vi "Teleop.vi"(10 "Match Info":T1={"Autonomous Elapsed Seconds"=0.0, "TeleOp Elapsed Seconds"=0.0, "Disabled Elapsed Seconds"=0.0, "Visited Autonomous"=FALSE, "Visited TeleOp"=FALSE, "Visited Disabled"=FALSE, "Autonomous Settings"={"Autonomous Style"=enum."Independent", "VI Refnum"=refnum}}, 11 "Call Context":T2) -> ()   [LabVIEW 2011]
doc: "This VI is called for each TeleOp packet received from the DS where the robot is not disabled. It is often used to read from the joysticks and update I/O or to update setpoints for timed control loops. It should complete and return within 20 milliseconds or it may miss DS packets."
uses:
  <vilib>/Rock Robotics/WPI/DriverStation/WPI_DriverStationDerivedRobotMode.ctl
  <vilib>/Rock Robotics/WPI/DriverStation/WPI_DriverStationMatch Info.ctl
  <vilib>/Rock Robotics/WPI/Relay/WPI_RelayValue.ctl
  <vilib>/Rock Robotics/WPI/DriverStation/DriverStationLCD/WPI_DriverStationLCDLCDLine.ctl
  Robot Global Data.vi
panel:
  in  "LDrive0":dbl
  in  "Rdrive0":dbl=0.9
  in  "Rdrive2":dbl=0.6
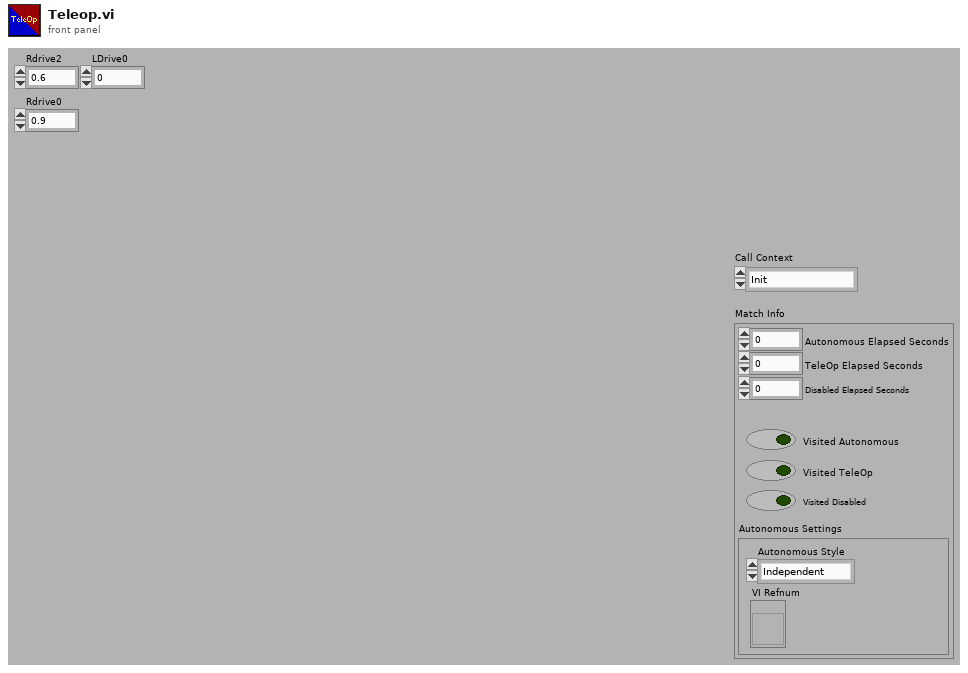
[diagram p1: front panel]
types:
  T1 = typedef "WPI_DriverStationMatch Info.ctl" = cluster{"Autonomous Elapsed Seconds":dbl, "TeleOp Elapsed Seconds":dbl, "Disabled Elapsed Seconds":dbl, "Visited Autonomous":bool, "Visited TeleOp":bool, "Visited Disabled":bool, "Autonomous Settings":cluster{"Autonomous Style":enum16{"Iterative", "Independent"}, "VI Refnum":refnum<vi>}}
  T2 = typedef "WPI_DriverStationDerivedRobotMode.ctl" = enum16{"Init", "Execute", "Stop"}
  T3 = typedef "WPI_RelayValue.ctl" = enum16{"Off", "On", "Forward", "Reverse"}
  T4 = typedef "WPI_JoystickDevRef.ctl" = cluster{"Device":T5}
  T5 = typedef "WPI_JoystickDeviceEnum.ctl" = enum16{"USB 1", "USB 2", "USB 3", "USB 4", "Kinect 1", "Kinect 2"}
  T6 = typedef "WPI_JoystickButtonState.ctl" = cluster{"Button 1":bool, "Button 2":bool, "Button 3":bool, "Button 4":bool, "Button 5":bool, "Button 6":bool, "Button 7":bool, "Button 8":bool, "Button 9":bool, "Button 10":bool, "Button 11":bool, "Button 12":bool}
  T7 = cluster{"axis 1 (x)":dbl, "axis 2 (y)":dbl, "axis 3 (throttle)":dbl, "axis 4":dbl, "axis 5":dbl, "axis 6":dbl}
  T8 = typedef "WPI_MotorControlDeviceRef.ctl" = cluster{"DeviceStatus":errorcluster, "Type":enum16{"PWM", "CAN"}, "PWM":cluster{"Digital Module":T9, "PWM Channel":T10, "DeadBand":T11}, "CAN":cluster{"Device Number":u8, "Control Mode":T12, "Semaphore":T13, "Max Vout":dbl}, "Invert":bool, "TransformRef":T14, "InvTransformRef":T14}
  T9 = typedef "FPGA_TypedefDigitalModule.ctl" = enum16{"Digital Module 1", "Digital Module 2"}
  T10 = typedef "FPGA_DIOPWMChannel.ctl" = enum8{"PWM 1", "PWM 2", "PWM 3", "PWM 4", "PWM 5", "PWM 6", "PWM 7", "PWM 8", "PWM 9", "PWM 10", "Invalid"}
  T11 = typedef "WPI_PWMDeadband.ctl" = cluster{"Name":string, "maxPositivePwm":i32, "minPositivePwm":i32, "centerPwm":i32, "maxNegativePwm":i32, "minNegativePwm":i32, "angularRange":u16}
  T12 = typedef "WPI_CANJaguar_ControlMode.ctl" = enum8{"Percent VBus", "Current", "Speed", "Position", "Voltage"}
  T13 = typedef "Semaphore RefNum" = refnum<k1>
  T14 = typedef "WPI_PWMTransform_ConPane.ctl" = refnum<vi>
  T15 = cluster{"Driver Station Digital Input (1-8)[0]":bool, "Driver Station Digital Input (1-8)[1]":bool, "Driver Station Digital Input (1-8)[2]":bool, "Driver Station Digital Input (1-8)[3]":bool, "Driver Station Digital Input (1-8)[4]":bool, "Driver Station Digital Input (1-8)[5]":bool, "Driver Station Digital Input (1-8)[6]":bool, "Driver Station Digital Input (1-8)[7]":bool, "Driver Station Digital Input (1-8)[8]":bool}
  T16 = typedef "WPI_RelayDevRef.ctl" = cluster{"DevStatus":errorcluster, "Relay Channel":T17, "Digital Module":T9, "Relay Direction":T18}
  T17 = typedef "FPGA_DIORelayChannel.ctl" = enum8{"Relay 1", "Relay 2", "Relay 3", "Relay 4", "Relay 5", "Relay 6", "Relay 7", "Relay 8", "Invalid"}
  T18 = typedef "WPI_RelayDirection.ctl" = enum16{"Both directions", "Forward only", "Reverse only"}
  T19 = typedef "WPI_DigitalInputDevRef.ctl" = cluster{"DevStatus":errorcluster, "DIO Channel":T20, "Digital Module":T9}
  T20 = typedef "FPGA_DIOChannel.ctl" = enum8{"DIO 1", "DIO 2", "DIO 3", "DIO 4", "DIO 5", "DIO 6", "DIO 7", "DIO 8", "DIO 9", "DIO 10", "DIO 11", "DIO 12", "DIO 13", "DIO 14", "Invalid"}
  T21 = typedef "WPI_EncoderDevRef.ctl" = cluster{"DevStatus":errorcluster, "EncoderIndex":T22, "CounterIndex":T23, "DistancePerCount":dbl, "Decoding Type":T24}
  T22 = typedef "FPGA_EncoderIdx.ctl" = enum8{"Enc 0", "Enc 1", "Enc 2", "Enc 3", "Invalid"}
  T23 = typedef "FPGA_CounterCtrSystemIndex.ctl" = enum8{"Ctr 0", "Ctr 1", "Ctr 2", "Ctr 3", "Ctr 4", "Ctr 5", "Ctr 6", "Ctr 7", "Invalid"}
  T24 = typedef "WPI_EncoderType.ctl" = enum16{"1x", "2x", "4x"}
  T25 = typedef "WPI_DriverStationLCDLCDLine.ctl" = enum16{"Main - Line 1", "User - Line 2", "User - Line 3", "User - Line 4", "User - Line 5", "User - Line 6"}
  T26 = typedef "WPI_ServoDeviceRef.ctl" = cluster{"DeviceStatus":errorcluster, "Digital Module":T9, "PWM Channel":T10, "DeadBand":T11}
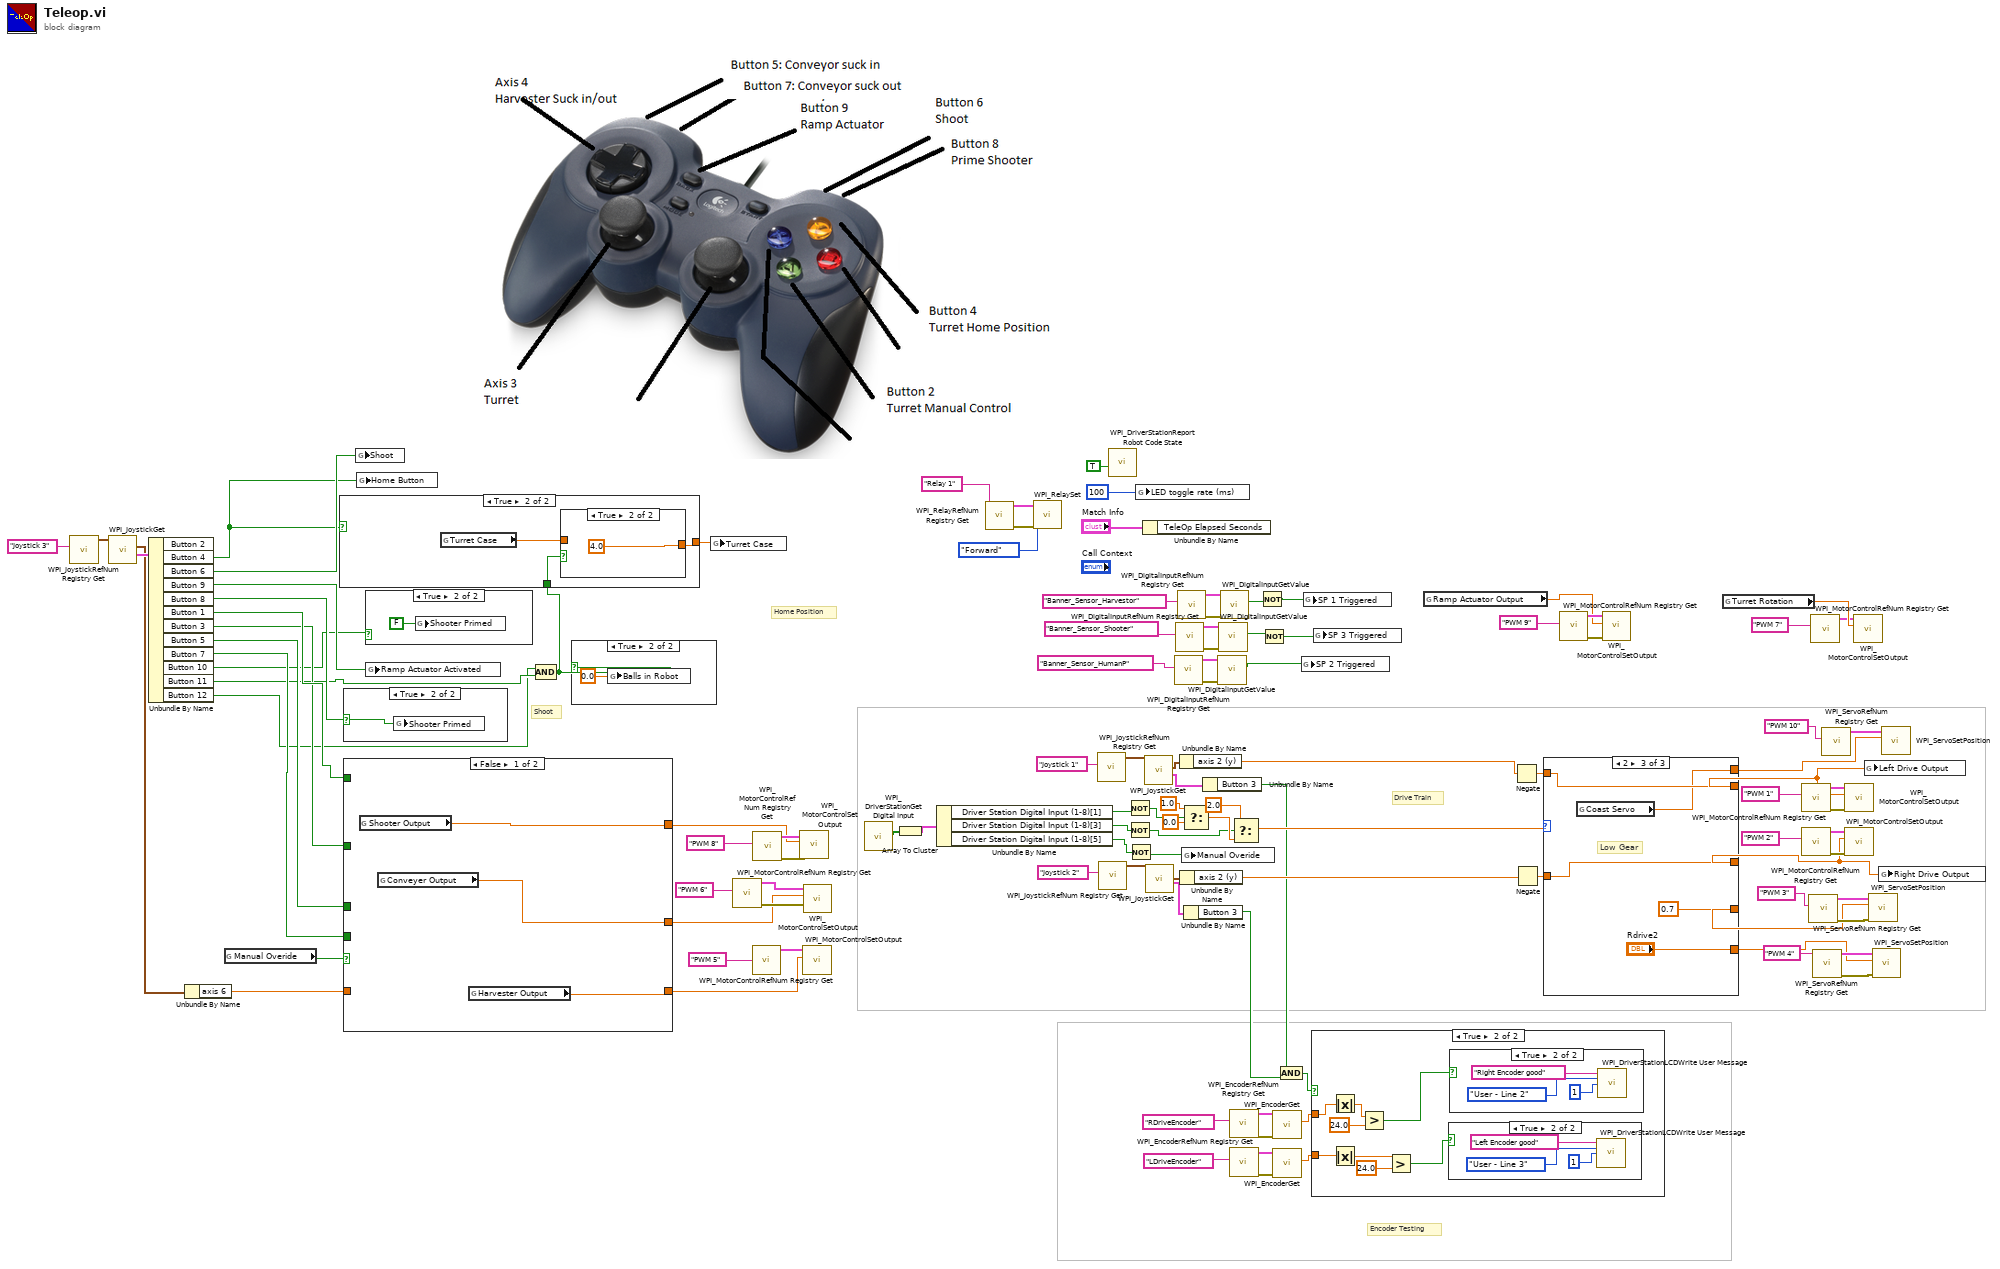
[diagram p0: block diagram]
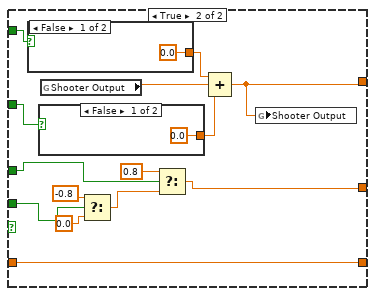
[diagram p7: hidden frame]
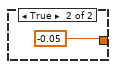
[diagram p8: hidden frame]
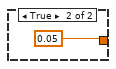
[diagram p9: hidden frame]
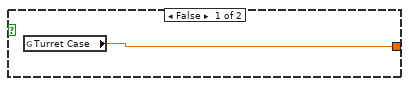
[diagram p11: hidden frame]
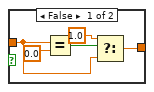
[diagram p12: hidden frame]
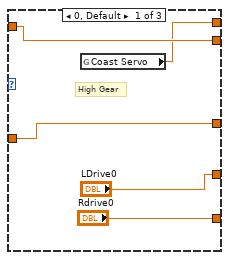
[diagram p13: hidden frame]
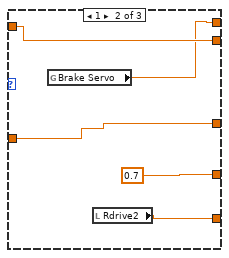
[diagram p14: hidden frame]
diagram:
  # "Encoder Testing"
  # "Shoot"
  # "Home Position"
  # "Drive Train"
  n1 = call <vilib>:"WPI_JoystickRefNum Registry Get.vi"("refnum name"="Joystick 3") -> ("JoystickDevRef"=w66:T4)  [unwired: 9 in, 1 out]
  n2 = call <vilib>:"WPI_JoystickGet.vi"("JoystickDevRef"=w66) -> ("Buttons"=w67:T6, "Axes"=w40:T7)  [unwired: 4 in, 1 out]
  n3 = Unbundle By Name(w67) -> ("Button 4"=w25:bool, "Button 6"=w65:bool, "Button 9"=w69:bool, "Button 8"=w41:bool, "Button 1"=w27:bool, "Button 3"=w26:bool, "Button 5"=w35:bool, "Button 7"=w34:bool, "Button 10"=w24:bool, "Button 11"=w23:bool, "Button 12"=w22:bool)  [unwired: 1 out]
  n4 = Unbundle By Name(w40) -> ("axis 6"=w20:dbl)
  n5 = global read "Robot Global Data.vi" "Manual Overide"() -> (w29:bool)
  n6 = case shown="True" w41 {
    selector: w41 -> [_ w114]
    frame False {
    }
    frame True {
      n7 = global write "Robot Global Data.vi" "Shooter Primed"(w114) -> ()
    }
  }
  n8 = case shown="False" w29 {
    tunnel: [w117 w119] -> w36
    tunnel: w27 -> [_ w124]
    tunnel: w26 -> [_ w123]
    tunnel: w35 -> [_ w126]
    tunnel: w34 -> [_ w127]
    tunnel: [w116 w125] -> w30
    tunnel: [w115 w118] -> w21
    tunnel: w20 -> [_ w118]
    frame False {
      n9 = global read "Robot Global Data.vi" "Shooter Output"() -> (w117:dbl)
      n10 = global read "Robot Global Data.vi" "Conveyer Output"() -> (w116:dbl)
      n11 = global read "Robot Global Data.vi" "Harvester Output"() -> (w115:dbl)
    }
    frame True {
      n12 = case shown="False" w124 {
        tunnel: [0.0 0.05] -> w122
        frame False {
        }
        frame True {
        }
      }
      n13 = case shown="False" w123 {
        tunnel: [0.0 -0.05] -> w121
        frame False {
        }
        frame True {
        }
      }
      n14 = global read "Robot Global Data.vi" "Shooter Output"() -> (w120:dbl)
      n15 = Select(t=-0.8, s=w127, f=0.0) -> (s? t:f=w131:dbl)
      n16 = Select(t=0.8, s=w126, f=w131) -> (s? t:f=w125:dbl)
      n17 = Compound Arithmetic op=ADD(w122, w120, w121) -> (w119:dbl)
      n18 = global write "Robot Global Data.vi" "Shooter Output"(w119) -> ()
    }
  }
  n19 = global write "Robot Global Data.vi" "Shoot"(w65) -> ()
  n20 = global write "Robot Global Data.vi" "Home Button"(w25) -> ()
  n21 = case shown="True" w24 {
    frame False {
    }
    frame True {
      n22 = global write "Robot Global Data.vi" "Shooter Primed"(FALSE ("Shooter Primed")) -> ()
    }
  }
  n23 = global write "Robot Global Data.vi" "Ramp Actuator Activated"(w69) -> ()
  n24 = Compound Arithmetic op=AND(w22, w23) -> (w19:bool)
  n25 = case shown="True" w25 {
    tunnel: [w137 w138] -> w18
    tunnel: w19 -> [_ w140]
    frame False {
      n26 = global read "Robot Global Data.vi" "Turret Case"() -> (w137:dbl)
    }
    frame True {
      n27 = global read "Robot Global Data.vi" "Turret Case"() -> (w139:dbl)
      n28 = case shown="True" w140 {
        tunnel: w139 -> [w142 _]
        tunnel: [w141 4.0 ("Turret Case")] -> w138
        frame False {
          n29 = Equal?(x=w142, y=0.0) -> (x = y?=w144:bool)
          n30 = Select(t=1.0, s=w144, f=w142) -> (s? t:f=w141:dbl)
        }
        frame True {
        }
      }
    }
  }
  n31 = case shown="True" w19 {
    frame False {
    }
    frame True {
      n32 = global write "Robot Global Data.vi" "Balls in Robot"(0.0 ("Balls in Robot")) -> ()
    }
  }
  n33 = global write "Robot Global Data.vi" "Turret Case"(w18) -> ()
  n34 = call <vilib>:"WPI_MotorControlRefNum Registry Get.vi"("refnum name"="PWM 6") -> ("error out"=w31:errorcluster, "MotorControlDevRef"=w32:T8)  [unwired: 9 in]
  n35 = call <vilib>:"WPI_MotorControlRefNum Registry Get.vi"("refnum name"="PWM 5") -> ("MotorControlDevRef"=w59:T8)  [unwired: 9 in, 1 out]
  n36 = call <vilib>:"WPI_MotorControlRefNum Registry Get.vi"("refnum name"="PWM 8") -> ("error out"=w43:errorcluster, "MotorControlDevRef"=w44:T8)  [unwired: 9 in]
  n37 = call <vilib>:"WPI_MotorControlSetOutput.vi"("error in (no error)"=w43, "Output"=w36, "MotorControlDevRef"=w44) -> ()  [unwired: 7 in, 2 out]
  n38 = call <vilib>:"WPI_MotorControlSetOutput.vi"("Output"=w21, "MotorControlDevRef"=w59) -> ()  [unwired: 8 in, 2 out]
  n39 = call <vilib>:"WPI_MotorControlSetOutput.vi"("error in (no error)"=w31, "Output"=w30, "MotorControlDevRef"=w32) -> ()  [unwired: 7 in, 2 out]
  n40 = call <vilib>:"WPI_DriverStationGet Digital Input.vi"() -> ("Driver Station Digital Input (1-8)"=w88:bool[])  [unwired: 11 in]
  n41 = Array To Cluster(array=w88) -> (cluster=w110:T15)
  n42 = Unbundle By Name(w110) -> ("Driver Station Digital Input (1-8)[1]"=w91:bool, "Driver Station Digital Input (1-8)[3]"=w90:bool, "Driver Station Digital Input (1-8)[5]"=w37:bool)
  n43 = call <vilib>:"WPI_RelayRefNum Registry Get.vi"("refnum name"="Relay 1") -> ("error out"=w63:errorcluster, "RelayDevRef"=w64:T16)  [unwired: 9 in]
  n44 = call <vilib>:"WPI_RelaySet.vi"("error in (no error)"=w63, "RelayValue"=WPI_RelayValue."Forward", "RelayDevRef"=w64) -> ()  [unwired: 7 in, 2 out]
  n45 = call <vilib>:"WPI_JoystickRefNum Registry Get.vi"("refnum name"="Joystick 1") -> ("JoystickDevRef"=w103:T4)  [unwired: 9 in, 1 out]
  n46 = call <vilib>:"WPI_JoystickRefNum Registry Get.vi"("refnum name"="Joystick 2") -> ("JoystickDevRef"=w101:T4)  [unwired: 9 in, 1 out]
  n47 = call <vilib>:"WPI_DriverStationReport Robot Code State.vi"("TeleOp"=TRUE ("Autonomous")) -> ()  [unwired: 10 in, 1 out]
  n48 = Not(x=w91) -> (.not. x?=w89:bool)
  n49 = Not(x=w90) -> (.not. x?=w39:bool)
  n50 = Not(x=w37) -> (.not. x?=w38:bool)
  n51 = global write "Robot Global Data.vi" "LED toggle rate (ms)"(u32 100 ("LED ms toggle rate")) -> ()
  n52 = Unbundle By Name("Match Info") -> ()  [unwired: 1 out]
  n53 = call <vilib>:"WPI_JoystickGet.vi"("JoystickDevRef"=w103) -> ("Buttons"=w15:T6, "Axes"=w16:T7)  [unwired: 4 in, 1 out]
  n54 = call <vilib>:"WPI_JoystickGet.vi"("JoystickDevRef"=w101) -> ("Buttons"=w17:T6, "Axes"=w102:T7)  [unwired: 4 in, 1 out]
  n55 = call <vilib>:"WPI_DigitalInputRefNum Registry Get.vi"("refnum name"="Banner_Sensor_HumanP") -> ("error out"=w54:errorcluster, "DigitalInputDevRef"=w53:T19)  [unwired: 9 in]
  n56 = call <vilib>:"WPI_DigitalInputRefNum Registry Get.vi"("refnum name"="Banner_Sensor_Shooter") -> ("error out"=w55:errorcluster, "DigitalInputDevRef"=w56:T19)  [unwired: 9 in]
  n57 = call <vilib>:"WPI_DigitalInputRefNum Registry Get.vi"("refnum name"="Banner_Sensor_Harvestor") -> ("error out"=w58:errorcluster, "DigitalInputDevRef"=w57:T19)  [unwired: 9 in]
  n58 = Unbundle By Name(w16) -> ("axis 2 (y)"=w87:dbl)
  n59 = Unbundle By Name(w102) -> ("axis 2 (y)"=w85:dbl)
  n60 = Select(t=1.0, s=w89, f=0.0 ("t")) -> (s? t:f=w107:dbl)
  n61 = global write "Robot Global Data.vi" "Manual Overide"(w38) -> ()
  n62 = Unbundle By Name(w17) -> ("Button 3"=w13:bool)
  n63 = Unbundle By Name(w15) -> ("Button 3"=w14:bool)
  n64 = call <vilib>:"WPI_DigitalInputGetValue.vi"("error in (no error)"=w54, "DigitalInputDevRef"=w53) -> ("Value"=w49:bool)  [unwired: 7 in, 2 out]
  n65 = call <vilib>:"WPI_DigitalInputGetValue.vi"("error in (no error)"=w55, "DigitalInputDevRef"=w56) -> ("Value"=w48:bool)  [unwired: 7 in, 2 out]
  n66 = call <vilib>:"WPI_DigitalInputGetValue.vi"("error in (no error)"=w58, "DigitalInputDevRef"=w57) -> ("Value"=w46:bool)  [unwired: 7 in, 2 out]
  n67 = call <vilib>:"WPI_EncoderRefNum Registry Get.vi"("refnum name"="RDriveEncoder") -> ("error out"=w9:errorcluster, "EncoderDevRef"=w10:T21)  [unwired: 9 in]
  n68 = call <vilib>:"WPI_EncoderRefNum Registry Get.vi"("refnum name"="LDriveEncoder") -> ("error out"=w8:errorcluster, "EncoderDevRef"=w7:T21)  [unwired: 9 in]
  n69 = Select(t=2.0, s=w39, f=w107) -> (s? t:f=w105:dbl)
  n70 = Not(x=w46) -> (.not. x?=w45:bool)
  n71 = Not(x=w48) -> (.not. x?=w47:bool)
  n72 = call <vilib>:"WPI_EncoderGet.vi"("error in (no error)"=w9, "EncoderDevRef"=w10) -> ("Distance"=w5:dbl)  [unwired: 4 in, 5 out]
  n73 = call <vilib>:"WPI_EncoderGet.vi"("error in (no error)"=w8, "EncoderDevRef"=w7) -> ("Distance"=w4:dbl)  [unwired: 4 in, 5 out]
  n74 = And(x=w14, y=w13) -> (x .and. y?=w12:bool)
  n75 = global write "Robot Global Data.vi" "SP 2 Triggered"(w49) -> ()
  n76 = global write "Robot Global Data.vi" "SP 1 Triggered"(w45) -> ()
  n77 = case shown="True" w12 {
    tunnel: w5 -> [_ w150]
    tunnel: w4 -> [_ w149]
    frame False {
    }
    frame True {
      n78 = Absolute Value(x=w150) -> (abs(x)=w151:dbl)
      n79 = Absolute Value(x=w149) -> (abs(x)=w148:dbl)
      n80 = Greater?(x=w151, y=24.0) -> (0:w154:bool)
      n81 = Greater?(x=w148, y=24.0) -> (0:w152:bool)
      n82 = case shown="True" w152 {
        frame False {
        }
        frame True {
          n83 = call <vilib>:"WPI_DriverStationLCDWrite User Message.vi"("line text"="Left Encoder good", "line"=WPI_DriverStationLCDLCDLine."User - Line 3", "starting column"=i8 1) -> ()  [unwired: 2 in, 11 out]
        }
      }
      n84 = case shown="True" w154 {
        frame False {
        }
        frame True {
          n85 = call <vilib>:"WPI_DriverStationLCDWrite User Message.vi"("line text"="Right Encoder good", "line"=WPI_DriverStationLCDLCDLine."User - Line 2", "starting column"=i8 1) -> ()  [unwired: 2 in, 11 out]
        }
      }
    }
  }
  n86 = global write "Robot Global Data.vi" "SP 3 Triggered"(w47) -> ()
  n87 = global read "Robot Global Data.vi" "Ramp Actuator Output"() -> (w28:dbl)
  n88 = Negate(x=w87) -> (-x=w86:dbl)
  n89 = Negate(x=w85) -> (-x=w84:dbl)
  n90 = case shown="2" w105 {
    tunnel: w84 -> [w166 w169 w176]
    tunnel: [w166 w169 w176] -> w76
    tunnel: [w165 w168 w175] -> w77
    tunnel: ["LDrive0" 0.7 0.7] -> w93
    tunnel: ["Rdrive0" w170 "Rdrive2"] -> w92
    tunnel: w86 -> [w165 w168 w175]
    tunnel: [w162 w167 w172] -> w1
    frame 0, Default {
      # "High Gear"
      n91 = global read "Robot Global Data.vi" "Coast Servo"() -> (w162:dbl)
    }
    frame 1 {
      n92 = global read "Robot Global Data.vi" "Brake Servo"() -> (w167:dbl)
      n93 = local read "Rdrive2"() -> (w170:dbl)
    }
    frame 2 {
      # "Low Gear"
      n94 = global read "Robot Global Data.vi" "Coast Servo"() -> (w172:dbl)
    }
  }
  n95 = call <vilib>:"WPI_MotorControlRefNum Registry Get.vi"("refnum name"="PWM 9") -> ("error out"=w74:errorcluster, "MotorControlDevRef"=w73:T8)  [unwired: 9 in]
  n96 = call <vilib>:"WPI_MotorControlSetOutput.vi"("error in (no error)"=w74, "Output"=w28, "MotorControlDevRef"=w73) -> ()  [unwired: 7 in, 2 out]
  n97 = global read "Robot Global Data.vi" "Turret Rotation"() -> (w72:dbl)
  n98 = call <vilib>:"WPI_MotorControlRefNum Registry Get.vi"("refnum name"="PWM 1") -> ("error out"=w81:errorcluster, "MotorControlDevRef"=w83:T8)  [unwired: 9 in]
  n99 = call <vilib>:"WPI_MotorControlRefNum Registry Get.vi"("refnum name"="PWM 2") -> ("error out"=w80:errorcluster, "MotorControlDevRef"=w79:T8)  [unwired: 9 in]
  n100 = call <vilib>:"WPI_ServoRefNum Registry Get.vi"("refnum name"="PWM 3") -> ("error out"=w97:errorcluster, "ServoDeviceRef"=w98:T26)  [unwired: 9 in]
  n101 = call <vilib>:"WPI_MotorControlRefNum Registry Get.vi"("refnum name"="PWM 7") -> ("MotorControlDevRef"=w70:T8)  [unwired: 9 in, 1 out]
  n102 = call <vilib>:"WPI_ServoRefNum Registry Get.vi"("refnum name"="PWM 4") -> ("error out"=w96:errorcluster, "ServoDeviceRef"=w95:T26)  [unwired: 9 in]
  n103 = call <vilib>:"WPI_ServoRefNum Registry Get.vi"("refnum name"="PWM 10") -> ("ServoDeviceRef"=w3:T26)  [unwired: 9 in, 1 out]
  n104 = call <vilib>:"WPI_MotorControlSetOutput.vi"("error in (no error)"=w81, "Output"=w77, "MotorControlDevRef"=w83) -> ()  [unwired: 7 in, 2 out]
  n105 = call <vilib>:"WPI_MotorControlSetOutput.vi"("error in (no error)"=w80, "Output"=w76, "MotorControlDevRef"=w79) -> ()  [unwired: 7 in, 2 out]
  n106 = call <vilib>:"WPI_MotorControlSetOutput.vi"("Output"=w72, "MotorControlDevRef"=w70) -> ()  [unwired: 8 in, 2 out]
  n107 = global write "Robot Global Data.vi" "Left Drive Output"(w77) -> ()
  n108 = call <vilib>:"WPI_ServoSetPosition.vi"("error in (no error)"=w97, "Position"=w93, "ServoDeviceRef"=w98) -> ()  [unwired: 7 in, 2 out]
  n109 = call <vilib>:"WPI_ServoSetPosition.vi"("error in (no error)"=w96, "Position"=w92, "ServoDeviceRef"=w95) -> ()  [unwired: 7 in, 2 out]
  n110 = global write "Robot Global Data.vi" "Right Drive Output"(w76) -> ()
  n111 = call <vilib>:"WPI_ServoSetPosition.vi"("Position"=w1, "ServoDeviceRef"=w3) -> ()  [unwired: 8 in, 2 out]
